vi "74HC138功能测试.vi"(0 "A0":bool, 1 "A1":bool, 2 "A2":bool, 5 "S1":bool, 6 "S2`":bool, 7 "S3`":bool) -> (20 "Y0`":bool, 21 "Y1`":bool, 22 "Y2`":bool, 23 "Y3`":bool, 24 "Y4`":bool, 25 "Y5`":bool, 26 "Y6`":bool, 27 "Y7`":bool)   [LabVIEW 2018]
panel:
  in  "结束":bool
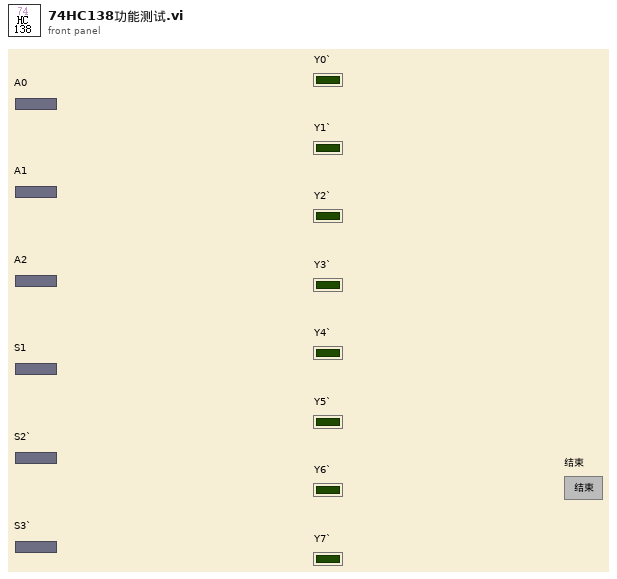
[diagram p1: front panel]
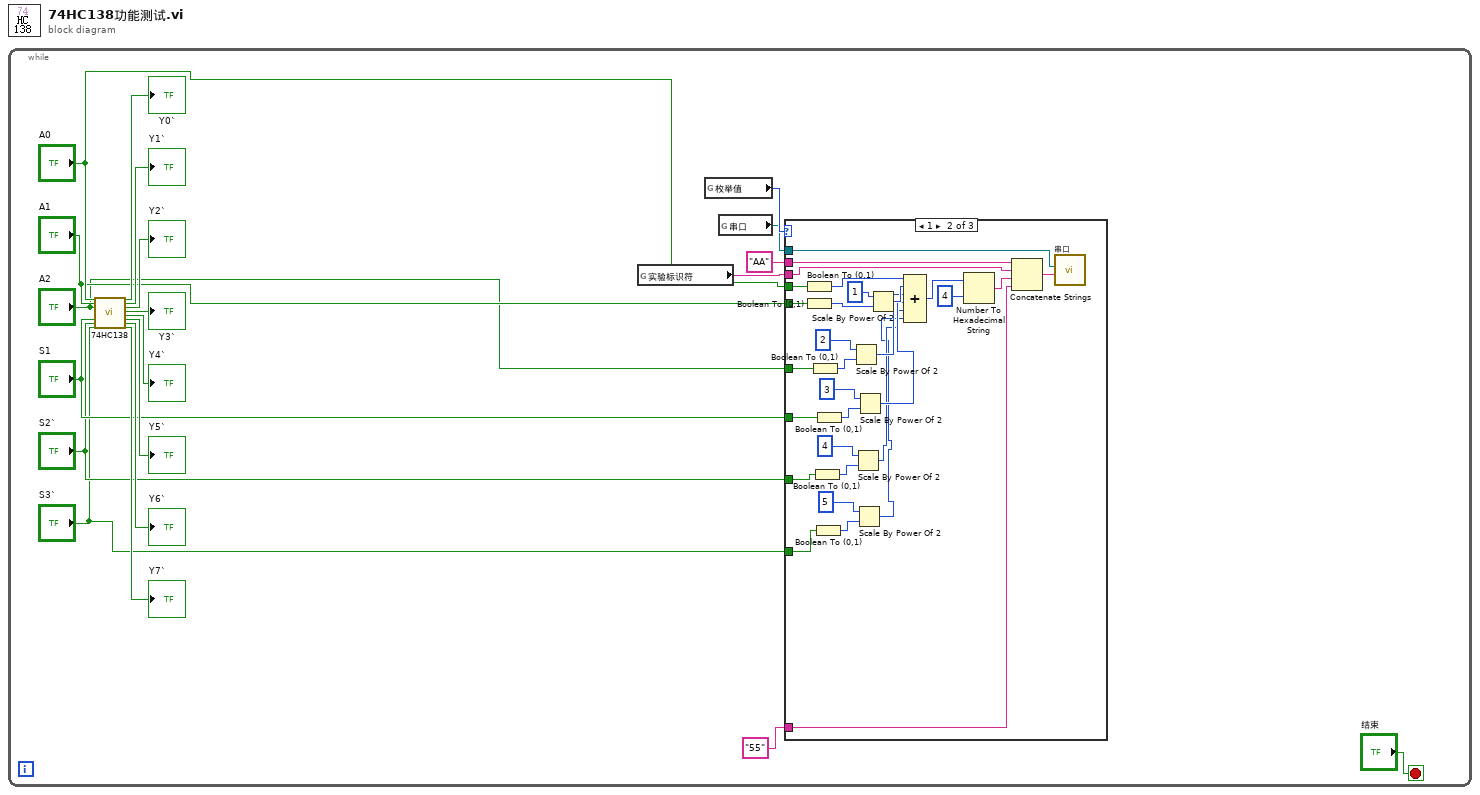
[diagram p0: block diagram]
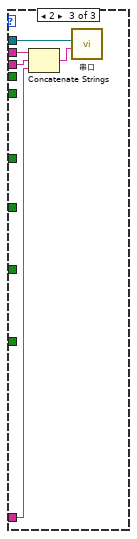
[diagram p3: hidden frame]
diagram:
  n1 = while {
    stop <- "结束" stop-if-true
    n2 = call "74HC138.vi"("A0"="A0", "A1"="A1", "A2"="A2", "S1"="S1", "S2`"="S2`", "S3`"="S3`") -> ("Y0`"=→"Y0`":bool, "Y1`"=→"Y1`":bool, "Y2`"=→"Y2`":bool, "Y3`"=→"Y3`":bool, "Y4`"=→"Y4`":bool, "Y5`"=→"Y5`":bool, "Y6`"=→"Y6`":bool, "Y7`"=→"Y7`":bool)  [unwired: 14 in]
    n3 = global read "全局变量.vi" "实验标识符"() -> (w9:string)
    n4 = global read "全局变量.vi" "枚举值"() -> (w11:i8)
    n5 = global read "全局变量.vi" "串口"() -> (w10:refnum<visa-resource-name>)
    n6 = case shown="1" w11 {
      tunnel: "A0" -> [_ w45 _]
      tunnel: w10 -> [_ w44 w53]
      tunnel: w9 -> [_ w43 w54]
      tunnel: "55" -> [_ w42 w51]
      tunnel: "AA" -> [_ w41 w52]
      tunnel: "A1" -> [_ w25 _]
      tunnel: "A2" -> [_ w24 _]
      tunnel: "S1" -> [_ w23 _]
      tunnel: "S2`" -> [_ w22 _]
      tunnel: "S3`" -> [_ w21 _]
      frame 0, Default {
      }
      frame 1 {
        n7 = Boolean To (0,1)(Boolean=w45) -> (0, 1=w49:i16)
        n8 = Boolean To (0,1)(Boolean=w25) -> (0, 1=w47:i16)
        n9 = Boolean To (0,1)(Boolean=w24) -> (0, 1=w36:i16)
        n10 = Boolean To (0,1)(Boolean=w22) -> (0, 1=w32:i16)
        n11 = Boolean To (0,1)(Boolean=w21) -> (0, 1=w30:i16)
        n12 = Boolean To (0,1)(Boolean=w23) -> (0, 1=w34:i16)
        n13 = Scale By Power Of 2(n=2, x=w36) -> (x*2^n=w37:i16)
        n14 = Scale By Power Of 2(n=4, x=w32) -> (x*2^n=w27:i16)
        n15 = Scale By Power Of 2(n=5, x=w30) -> (x*2^n=w26:i16)
        n16 = Scale By Power Of 2(n=3, x=w34) -> (x*2^n=w28:i16)
        n17 = Scale By Power Of 2(n=1, x=w47) -> (x*2^n=w48:i16)
        n18 = Compound Arithmetic op=ADD ("复合运算")(w49, w48, w37, w28, w27, w26) -> (w40:i16)
        n19 = Number To Hexadecimal String(1:4, 2:w40) -> (0:w38:string)
        n20 = Concatenate Strings(w41, w43, w38, w42) -> (w50:string)
        n21 = call "串口.vi"("字符串"=w50, "VISA resource name"=w44) -> ()  [unwired: 10 in]
      }
      frame 2 {
        n22 = Concatenate Strings(w52, w54, w51) -> (w55:string)
        n23 = call "串口.vi"("字符串"=w55, "VISA resource name"=w53) -> ()  [unwired: 10 in]
      }
    }
  }
